vi "校准日志.vi"(8 "error in (no error)":errorcluster, 10 "table":string="操作日志", 11 "日志信息":string) -> (0 "error out":errorcluster)   [LabVIEW 2016, in "斯坦道多参数.lvlib"]
uses:
  <vilib>/addons/database/Auxilliary.llb/DB Tools Transaction.ctl
  <vilib>/addons/database/Auxilliary.llb/DB Tools Isolation Level.ctl
  <vilib>/Utility/sysdir.llb/System Directory Type.ctl
  <vilib>/addons/database/Connection.llb/DB Tools Open Connec (String).vi
  <vilib>/addons/database/Connection.llb/Conn Transaction.vi
  <vilib>/addons/database/NI_Database_API.lvlib
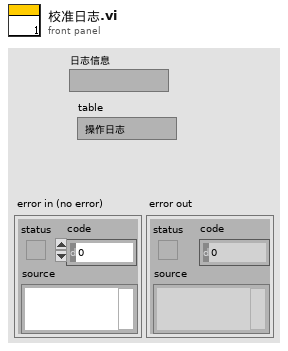
[diagram p1: front panel]
types:
  T1 = typedef "NI_Database_API.lvlib/DB Tools Isolation Level.ctl" = enum16{"chaos", "read uncommitted", "read committed", "repeatable read", "serializable"}
  T2 = typedef "NI_Database_API.lvlib/DB Tools Transaction.ctl" = enum16{"begin", "commit", "rollback"}
  T3 = cluster{"时间标识":timestamp, "设备":string, "日志信息":string, "流程参数":string}
  T4 = typedef "System Directory Type.ctl" = i32
  T5 = typedef "NI_Database_API.lvlib/Conn ObjectReference.ctl" = refnum<k1>
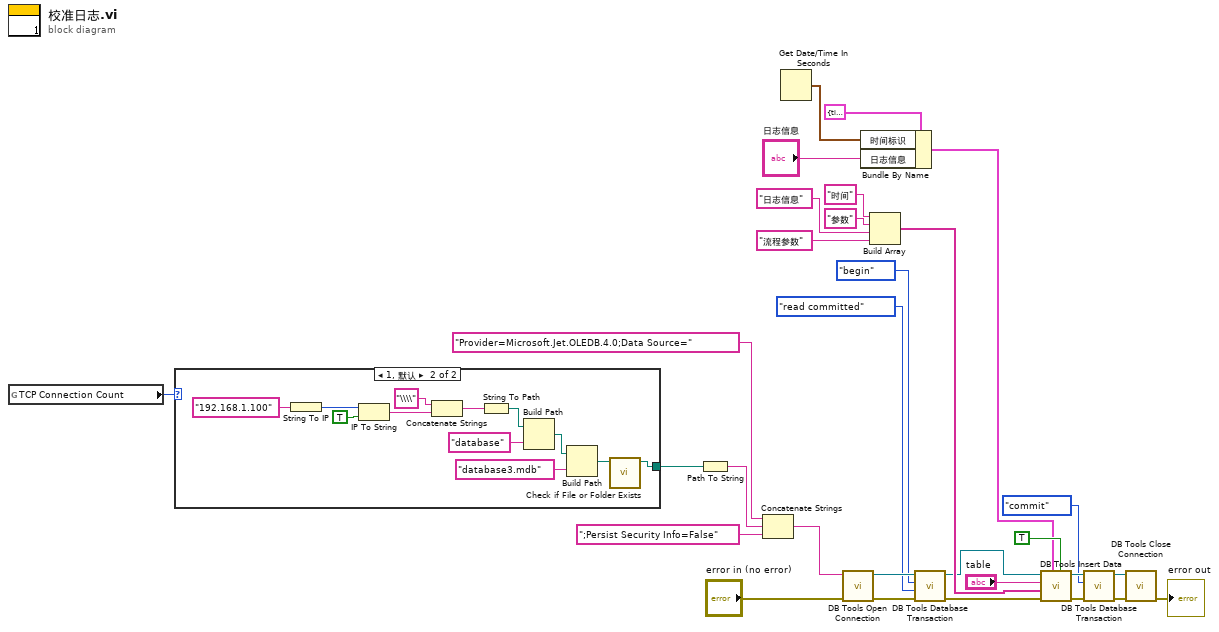
[diagram p0: block diagram]
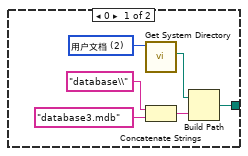
[diagram p2: hidden frame]
diagram:
  n1 = global read "多参数全局变量.vi" "TCP Connection Count"() -> (w1:u32)
  n2 = case shown="1, 默认" w1 {
    tunnel: [w31 w37] -> w4
    frame 0 {
      w32 = T4 2 items=["用户目录"=0, "用户桌面"=1, "用户文档"=2, "用户应用程序数据"=3, "用户设置"=4, "用户临时目录"=5, "公共文档"=6, "公共应用程序数据"=7, "公共设置"=8, "公共缓存"=13, "系统核心库"=9, "系统安装库"=10, "应用程序文件"=11, "启动盘根目录"=12] ("system directory type")
      n3 = call <vilib>:"Get System Directory.vi"("system directory type"=w32) -> ("system directory"=w33:path)  [unwired: 10 in]
      n4 = Concatenate Strings("database\\" ("condition"), "database3.mdb" ("database")) -> (w35:string)
      n5 = Build Path(base path=w33, name or relative path=w35) -> (appended path=w31:path)
    }
    frame 1, Default {
      n6 = String To IP(1:"192.168.1.100" ("名称")) -> (0:w38:u32)
      n7 = IP To String(1:TRUE ("句点符号？(F)"), 2:w38) -> (0:w44:string)
      n8 = Concatenate Strings("\\\\" ("字符串"), w44) -> (w41:string)
      n9 = String To Path(string=w41) -> (path=w39:path)
      n10 = Build Path(base path=w39, name or relative path="database" ("名称或相对路径")) -> (appended path=w43:path)
      n11 = Build Path(base path=w43, name or relative path="database3.mdb" ("database")) -> (appended path=w45:path)
      n12 = call <vilib>:"Check if File or Folder Exists.vi"("path"=w45) -> ("dup path"=w37:path)  [unwired: 8 in, 2 out]
    }
  }
  n13 = Path To String(path=w4) -> (string=w24:string)
  n14 = Concatenate Strings("Provider=Microsoft.Jet.OLEDB.4.0;Data Source=" ("condition"), w24, ";Persist Security Info=False" ("condition")) -> (w22:string)
  n15 = Get Date/Time In Seconds() -> (seconds since 1Jan1904=w17:timestamp)
  n16 = call-poly <vilib>:"DB Tools Open Connection.vi"("error in (no error)"="error in (no error)", "connection information"=w22) -> ("error out"=w13:errorcluster, "connection reference"=w21:T5)  [unwired: 6 in]
  n17 = Bundle By Name(cluster=T3 {"时间标识"=timestamp(0 s since 1904-01-01), "设备"="多参数", "日志信息"="", "流程参数"=""} ("data in"), "时间标识"=w17, "日志信息"="日志信息") -> (w16:T3)
  n18 = Build Array("时间", "参数" ("元素"), "日志信息", "流程参数") -> (w19:string[])
  n19 = call-poly <vilib>:"DB Tools Database Transaction.vi"("error in (no error)"=w13, "isolation level (chaos)"=DB_Tools_Isolation_Level."read committed", "operation (begin)"=DB_Tools_Transaction."begin", "connection reference"=w21) -> ("error out"=w12:errorcluster, "connection reference out"=w14:T5)  [unwired: 2 in]
  n20 = call <vilib>:"DB Tools Insert Data.vi"("create table? (F)"=TRUE, "data"=w16, "error in (no error)"=w12, "columns"=w19, "table"="table", "connection reference"=w14) -> ("error out"=w9:errorcluster, "connection reference out"=w11:T5)  [unwired: 4 in]
  n21 = call-poly <vilib>:"DB Tools Database Transaction.vi"("error in (no error)"=w9, "operation (begin)"=DB_Tools_Transaction."commit", "connection reference"=w11) -> ("error out"=w8:errorcluster, "connection reference out"=w10:T5)  [unwired: 3 in]
  n22 = call <vilib>:"DB Tools Close Connection.vi"("error in (no error)"=w8, "connection reference"=w10) -> ("error out"=→"error out":errorcluster)  [unwired: 5 in]
